vi "Initialize Attributre-Parameter Map.vi"(8 "vs channel index":i32, 9 "dataType":string, 10 "parameterHandle":u64, 11 "Map in":map{u64, T1}(c390)) -> (3 "Map out":map{u64, T1}(c390))   [LabVIEW 2019, in "HLA Custom Device Engine.lvlib"]
uses:
  HLA Custom Device Engine.lvlib
  _typedefs/map_attr_param_data.ctl
  <vilib>/Utility/miscctls.llb/LVMapReplaceAction.ctl
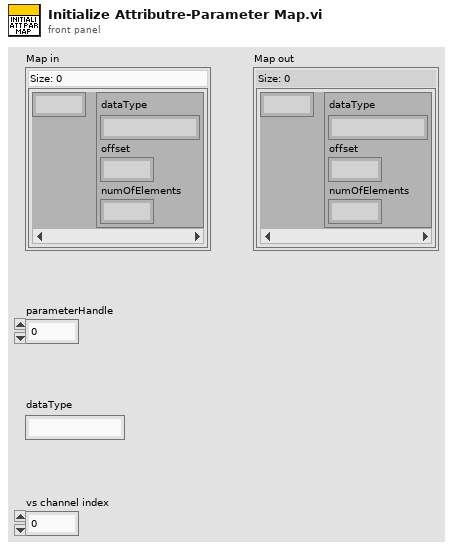
[diagram p1: front panel]
types:
  T1 = typedef "HLA Custom Device Engine.lvlib/map_attr_param_data.ctl" = cluster{"dataType":string, "offset":i32, "numOfElements":i32}
  T2 = typedef "LVMapReplaceAction.ctl" = enum32{"Modify Entry only if found", "Add or Modify Entry", "Delete Entry"}
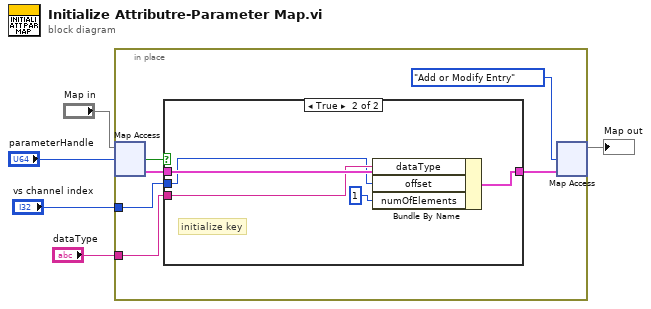
[diagram p0: block diagram]
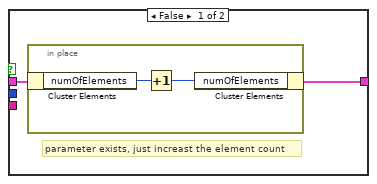
[diagram p2: hidden frame]
diagram:
  n1 = in-place {
    in-place-border: "dataType" -> [w9]
    in-place-border: "vs channel index" -> [w8]
    n2 = in-place-map #1("Map in", "parameterHandle") -> (w10:T1, w11:bool)  [unwired: 1 in]
    n3 = case shown="True" w11 {
      tunnel: w10 -> [w13 w20]
      tunnel: w9 -> [_ w19]
      tunnel: w8 -> [_ w18]
      tunnel: [w12 w16] -> w7
      frame False {
        # "parameter exists, just increast the element count"
        n4 = in-place {
          n5 = in-place-cluster #2(w13) -> ("numOfElements"=w15:i32)
          n6 = Increment(x=w15) -> (x+1=w14:i32)
          n7 = in-place-cluster #2("numOfElements"=w14) -> (w12:T1)
        }
      }
      frame True {
        # "initialize key"
        n8 = Bundle By Name(cluster=w20, "dataType"=w19, "offset"=w18, "numOfElements"=1) -> (w16:T1)
      }
    }
    n9 = in-place-map #1(w7, LVMapReplaceAction."Add or Modify Entry" ("action")) -> (→"Map out":map{u64, T1})  [unwired: 2 out]
  }
